vi "Main Tclk.vi"() -> ()   [LabVIEW 2018] (continued)
                        n5203 = local write "Status message"("Scanning FIB vertically to obtain beam profile" ("Status message")) -> ()
                        n5204 = Get Date/Time In Seconds() -> (seconds since 1Jan1904=w4280:timestamp)
                        n5205 = To Double Precision Float(number=w4280) -> (double precision float=w4279:dbl)
                        n5206 = property on="Measurements" class="WFChart (strict)"("History Data"=dbl[][] [], "XScale.Offset"=w4279) -> ()  [unwired: 2 in, 2 out]
                        n5207 = call "Wait to resume.vi"() -> ()  [unwired: 12 in]
                      }
                      frame #3 {
                        n5208 = local read "Logging status before profiling"() -> (w4306:bool)
                        n5209 = local write "FIB Profile"(FALSE ("FIB Profile")) -> ()
                        n5210 = local write "Enable logging"(w4306) -> ()
                      }
                    }
                  }
                }
              }
            }
          }
          event "Milling para": Value Change {
            n5211 = event-data() -> ()  [unwired: 2 out]
            n5212 = local read "Milling para"() -> (w4322:T35)
            n5213 = local read "FIB"() -> (w4328:bool)
            n5214 = case shown="True" w4328 {
              tunnel: [TRUE ("Origin") FALSE ("Origin")] -> w4329
              tunnel: [0.0 ("Y offset pre (um)") w4345] -> w4327
              frame False {
              }
              frame True {
                n5215 = local read "Y offset pre (um)"() -> (w4345:dbl)
              }
            }
            n5216 = Unbundle By Name(w4322) -> ("X size (um)"=w4337:sgl, "Z size (um)"=w4336:sgl, "Z-step (nm)"=w4308:dbl)
            n5217 = local write "SW error warning armed"(FALSE ("SW error warning armed")) -> ()
            n5218 = local write "Cycle time array"(u32[] [] ("Cycle time array")) -> ()
            n5219 = local write "Cycle time est offset array"(i16[] [] ("Cycle time array")) -> ()
            n5220 = expression code="x/1e3"(w4308) -> (w4334:dbl)
            n5221 = control-ref of="FIB Image"() -> (w4330:refnum<vi>)
            n5222 = local read "FIB Scan Parameters"() -> (w4321:T32)
            n5223 = local read "FIB Options"() -> (w4320:T33)
            n5224 = shared-variable ".\\Zeiss Library.lvlib\\Milling Z Voltage RT"() -> (w4319:sgl)  [unwired: 1 in, 1 out]
            n5225 = expression code="log2( x/0.1)"(w4337) -> (w4339:sgl)
            n5226 = Round Toward +Infinity(x=w4339) -> (ceil(x): smallest int >= x=w4341:sgl)
            n5227 = Scale By Power Of 2(n=w4341, x=ext 1.0) -> (x*2^n=w4338:ext)
            n5228 = Divide(x=w4336, y=w4334) -> (x/y=w4342:dbl)
            n5229 = Round To Nearest(number=w4342) -> (nearest integer value=w4331:dbl)
            n5230 = local read "Milling para"() -> (w4333:T35)
            n5231 = Increment(x=w4331) -> (x+1=w4332:dbl)
            n5232 = Multiply(x=w4331, y=w4334) -> (x*y=w4335:dbl)
            n5233 = Bundle By Name(cluster=w4333, "X resolution"=w4338, "Z resolution"=w4332, "Z size (um)"=w4335) -> (w4312:T35)
            n5234 = call "FIB image draw milling.vi"("Milling Z Voltage"=w4319, "Milling para"=w4312, "Z offset pre (um)"=w4327, "FIB Options"=w4320, "FIB Scan Parameters"=w4321, "Origin"=w4329, "Image reference"=w4330) -> ("X size factor"=w4310:dbl, "Trapezoidal"=w4309:cluster{"X":i16, "Y":i16}[])  [unwired: 3 in]
            n5235 = local write "Trapezoidal"(w4309) -> ()
            n5236 = control-ref of="Post Image"() -> (w4326:refnum<vi>)
            n5237 = local read "FIB Zoom Parameters"() -> (w4318:T34)
            n5238 = local write "Milling para"(w4312) -> ()
            n5239 = local read "X offset pre (um)"() -> (w4324:dbl)
            n5240 = local read "Y offset pre (um)"() -> (w4323:dbl)
            n5241 = call "FIB zoom image draw milling.vi"("Milling Z voltage"=w4319, "Milling para"=w4312, "Z offset pre (um)"=w4323, "X offset pre (um)"=w4324, "FIB Zoom Parameters"=w4318, "FIB Options"=w4320, "FIB Scan Parameters"=w4321, "Pre image"=FALSE, "Image reference"=w4326) -> ()  [unwired: 3 in]
            n5242 = Unbundle By Name(w4312) -> ("Line milling time (s)"=w4313:sgl, "Lines auto pause"=w4314:u16)
            n5243 = Compound Arithmetic op=MULTIPLY(w4313, w4314, w4310) -> (w4311:dbl)
            n5244 = local write "Milling time (s)"(w4311) -> ()
          }
          event "Milling para.Z-step (nm)": Value Change {
            n5245 = event-data() -> ()  [unwired: 7 out]
            n5246 = local read "Milling para"() -> (w4350:T35)
            n5247 = local read "FIB"() -> (w4351:bool)
            n5248 = case shown="True" w4351 {
              tunnel: [TRUE ("Origin") FALSE ("Origin")] -> w4352
              tunnel: [0.0 ("Y offset pre (um)") w4372] -> w4349
              frame False {
              }
              frame True {
                n5249 = local read "Y offset pre (um)"() -> (w4372:dbl)
              }
            }
            n5250 = Unbundle By Name(w4350) -> ("X size (um)"=w4363:sgl, "Z size (um)"=w4362:sgl, "Z-step (nm)"=w4347:dbl)
            n5251 = expression code="x/1e3"(w4347) -> (w4360:dbl)
            n5252 = control-ref of="FIB Image"() -> (w4356:refnum<vi>)
            n5253 = local read "FIB Scan Parameters"() -> (w4355:T32)
            n5254 = local read "FIB Options"() -> (w4354:T33)
            n5255 = shared-variable ".\\Zeiss Library.lvlib\\Milling Z Voltage RT"() -> (w4353:sgl)  [unwired: 1 in, 1 out]
            n5256 = expression code="log2( x/0.1)"(w4363) -> (w4365:sgl)
            n5257 = Round Toward +Infinity(x=w4365) -> (ceil(x): smallest int >= x=w4367:sgl)
            n5258 = call "FIB image draw milling.vi"("Milling Z Voltage"=w4353, "Milling para"=w4350, "Z offset pre (um)"=w4349, "FIB Options"=w4354, "FIB Scan Parameters"=w4355, "Origin"=w4352, "Image reference"=w4356) -> ()  [unwired: 3 in, 2 out]
            n5259 = Scale By Power Of 2(n=w4367, x=ext 1.0) -> (x*2^n=w4364:ext)
            n5260 = Divide(x=w4362, y=w4360) -> (x/y=w4368:dbl)
            n5261 = Round To Nearest(number=w4368) -> (nearest integer value=w4357:dbl)
            n5262 = local read "Milling para"() -> (w4359:T35)
            n5263 = Increment(x=w4357) -> (x+1=w4358:dbl)
            n5264 = Multiply(x=w4357, y=w4360) -> (x*y=w4361:dbl)
            n5265 = Round To Nearest(number=w4361) -> (nearest integer value=w4348:dbl)
            n5266 = Bundle By Name(cluster=w4359, "X resolution"=w4364, "Z resolution"=w4358, "Z size (um)"=w4348) -> (w4369:T35)
            n5267 = local write "Milling para"(w4369) -> ()
          }
          event "Milling para.Mill start from Last": Value Change {
            n5268 = event-data() -> ("NewVal"=w4374:bool)  [unwired: 6 out]
            n5269 = case shown="True" w4374 {
              frame False {
              }
              frame True {
                n5270 = stacked-sequence {
                  frame #0 {
                    n5271 = local read "Last milling snapshot"() -> (w4378:path)
                    n5272 = local read "Last FIB recipe"() -> (w4384:path)
                    n5273 = local read "Re-engage Files"() -> (w4390:path)
                    n5274 = File/Directory Info(path=w4384) -> (path out=w4383:path, error out=w4379:errorcluster)  [unwired: 1 in, 5 out]
                    n5275 = Build Path(base path=w4390, name or relative path="pre.png") -> (appended path=w4388:path)
                    n5276 = File/Directory Info(path=w4378) -> (path out=w4377:path, error out=w4375:errorcluster)  [unwired: 1 in, 5 out]
                    n5277 = Unbundle By Name(w4379) -> ("status"=w4380:bool)
                    n5278 = Unbundle By Name(w4375) -> ("status"=w4376:bool)
                    n5279 = File/Directory Info(path=w4388) -> (error out=w4385:errorcluster)  [unwired: 1 in, 6 out]
                    n5280 = case shown="False" w4376 {
                      tunnel: w4377 -> [w4394 _]
                      tunnel: [w4393 w4396] -> w4387
                      tunnel: w4375 -> [_ w4396]
                      frame False {
                        n5281 = call-poly <vilib>:"Read From XML File.vi"("XML File Path"=w4394) -> ("error out"=w4392:errorcluster, "XML Elements"=w4395:string)  [unwired: 8 in, 1 out]
                        n5282 = Unflatten From XML(xml string=w4395, type=T46 {"Timestamp"=timestamp(0 s since 1904-01-01), "Milling Z voltage"=0.0, "FIB slice #"=0, "Pause for reheat"=FALSE, "Last good FI"=0.0, "Focus index"=0.0, "SEM max FOV"=0.0, "Remaining X shift frames"=0, "Remaining Y shift frames"=0} ("output cluster"), error in (no error)=w4392) -> (error out=w4393:errorcluster)  [unwired: 1 out]
                      }
                      frame True {
                      }
                    }
                    n5283 = case shown="False" w4380 {
                      tunnel: [w4398 w4400] -> w4386
                      tunnel: w4383 -> [w4397 _]
                      tunnel: w4379 -> [_ w4400]
                      frame False {
                        n5284 = call "Recipe read write.vi"("Write"=FALSE, "Recipe path"=w4397) -> ("error out"=w4398:errorcluster)  [unwired: 6 in, 3 out]
                      }
                      frame True {
                      }
                    }
                    n5285 = Merge Errors(w4387, w4386, w4385) -> (w4381:errorcluster)
                    n5286 = Unbundle By Name(w4381) -> ("status"=w4382:bool)
                    n5287 = local write "error out"(w4381) -> ()
                    n5288 = case shown="True" w4382 {
                      frame False {
                      }
                      frame True {
                        n5289 = local read "Milling para"() -> (w4403:T35)
                        n5290 = Two Button Dialog(message="Files needed for resume do not exist or are corrupted\nLoad information from the last good data file (*.dat)?") -> (T button?=w4401:bool)  [unwired: 2 in]
                        "dat to csv and xml" <- w4401
                        n5291 = Bundle By Name(cluster=w4403, "Mill start from Last"=w4401) -> (w4402:T35)
                        n5292 = local write "Milling para"(w4402) -> ()
                      }
                    }
                  }
                  frame #1 {
                    n5293 = local read "dat to csv and xml"() -> (w4405:bool)
                    n5294 = case shown="True" w4405 {
                      frame False {
                      }
                      frame True {
                        n5295 = call "File Dialog4"("start path"=path "E:/Images", "prompt"="Select the last good .dat file", "pattern (all files)"="*.dat" ("pattern label"), "pattern label"="Data file") -> ("selected path"=w4408:path, "cancelled"=w4406:bool, "error out"=w4411:errorcluster)  [unwired: 8 in, 1 out]
                        n5296 = local write "Read recipe path"(w4408) -> ()
                        n5297 = local write "error out"(w4411) -> ()
                        n5298 = case shown="True" w4406 {
                          frame False {
                            n5299 = local write "Load recipe"(TRUE ("Load recipe")) -> ()
                          }
                          frame True {
                            n5300 = local read "Milling para"() -> (w4414:T35)
                            n5301 = Bundle By Name(cluster=w4414, "Mill start from Last"=FALSE) -> (w4416:T35)
                            n5302 = local write "Milling para"(w4416) -> ()
                          }
                        }
                      }
                    }
                  }
                  frame #2 {
                    n5303 = local read "Milling para"() -> (w4418:T35)
                    n5304 = Unbundle By Name(w4418) -> ("Mill start from Last"=w4417:bool)
                    n5305 = case shown="True" w4417 {
                      frame False {
                      }
                      frame True {
                        n5306 = One Button Dialog(message="Resume from the last recipe and milling position ") -> ()  [unwired: 1 in, 1 out]
                      }
                    }
                  }
                }
              }
            }
          }
          event "Milling para.FIB PID reset": Value Change {
            n5307 = event-data() -> ("NewVal"=w4420:bool)  [unwired: 2 out]
            n5308 = shared-variable ".\\Zeiss Library.lvlib\\FIB PID reset"(w4420) -> ()  [unwired: 1 in, 1 out]
          }
          event "Milling para.FIB PID target": Value Change {
            w4421 = FALSE ("FIB CL current alarm")
            n5309 = event-data() -> ()  [unwired: 7 out]
            n5310 = local write "Continued fine milling frames"(0 ("Continued fine milling frames")) -> ()
            n5311 = local read "Alert Settings"() -> (w4424:T36)
            n5312 = Bundle By Name(cluster=w4424, "FIB CL current alarm"=w4421, "Milling Z voltage alarm"=w4421) -> (w4423:T36)
            n5313 = local write "Alert Settings"(w4423) -> ()
          }
          event "Pre image": Value Change {
            n5314 = event-data() -> ("NewVal"=w4425:bool)  [unwired: 2 out]
            n5315 = case shown="True" w4425 {
              frame False {
                n5316 = local write "Status message"("standby" ("Status message")) -> ()
                n5317 = shared-variable "My Computer\\Zeiss Library.lvlib\\Realtime Imaging stop"(TRUE ("Unfreeze")) -> ()  [unwired: 1 in, 1 out]
              }
              frame True {
                n5318 = stacked-sequence {
                  frame #0 {
                    n5319 = local read "FIB HW Config"() -> (w4436:T23)
                    n5320 = local read "FIB HW Config"() -> (w4433:T23)
                    n5321 = local write "Status message"("FIB Pre Imaging" ("Status message")) -> ()
                    n5322 = Unbundle By Name(w4436) -> ("Beam blank"=w4435:tag)
                    n5323 = Unbundle By Name(w4433) -> ("FIB Ext Scan"=w4431:tag)
                    n5324 = local read "Api"() -> (w4428:refnum<k7>)
                    n5325 = call "FIB beam blank.vi"("ActiveX Container"=w4428, "Beam blanked"=TRUE, "lines"=w4435) -> ()  [unwired: 2 in, 1 out]
                    n5326 = call "FIB ext scan.vi"("Ext on"=TRUE ("data"), "FIB Ext Scan"=w4431) -> ()  [unwired: 9 in, 1 out]
                    n5327 = local write "Image Tabs"(T37."FIB Milling Offset after Pause" ("Image Tabs")) -> ()
                  }
                  frame #1 {
                    n5328 = local read "Machine Type"() -> (w4437:u8)
                    n5329 = case shown="1" w4437 {
                      frame 0, Default {
                      }
                      frame 1 {
                        w4440 = TRUE ("Close session")
                        n5330 = local read "COM port"() -> (w4442:refnum<visa-resource-name>)
                        n5331 = call "Remcon32 command.vi"("Initialization"=w4440, "SEM command"="edx 1", "COM port in"=w4442) -> ("COM port out"=w4441:refnum<visa-resource-name>)  [unwired: 5 in, 3 out]
                        n5332 = call "FIB mode.vi"("Close session"=w4440, "Iterations"=u32 3, "FIB mode"=T10."FIB", "COM port in"=w4441) -> ()  [unwired: 6 in, 2 out]
                      }
                    }
                  }
                  frame #2 {
                    n5333 = shared-variable ".\\Zeiss Library.lvlib\\Milling Z Voltage RT"() -> (w4445:sgl)  [unwired: 1 in, 1 out]
                    n5334 = local read "FIB Options"() -> (w4448:T33)
                    n5335 = local read "FIB Scan Parameters"() -> (w4452:T32)
                    n5336 = property on="Pre Image" class="IntGraph (strict)"() -> ("Width"=w4461:u32, "Height"=w4460:u32)  [unwired: 2 in, 2 out]
                    n5337 = local read "FIB Options"() -> (w4468:T33)
                    n5338 = local read "Milling para"() -> (w4451:T35)
                    n5339 = local read "FIB Scan Parameters"() -> (w4474:T32)
                    n5340 = expression code="x/1000"("FIB Y zoom pixel (nm)") -> (w4462:dbl)
                    n5341 = Decrement(x=w4460) -> (x-1=w4459:u32)
                    n5342 = Unbundle By Name(w4448) -> ("Flip z"=w4447:bool)
                    n5343 = Unbundle By Name(w4468) -> ("Flip x"=w4464:bool)
                    n5344 = Unbundle By Name(w4451) -> ("X offset (um)"=w4480:sgl, "X center (um)"=w4479:sgl, "FIB FOV (um)"=w4450:sgl)
                    n5345 = Multiply(x=w4462, y=w4459) -> (x*y=w4458:dbl)
                    "FIB Y zoom size (um)" <- w4458
                    n5346 = Unbundle By Name(w4452) -> ("Z size (V)"=w4453:dbl)
                    n5347 = Unbundle By Name(w4474) -> ("X size (V)"=w4469:dbl)
                    n5348 = Negate(x=w4445) -> (-x=w4446:sgl)
                    n5349 = Add(x=w4480, y=w4479) -> (x+y=w4481:sgl)
                    n5350 = Select(t=w4446, s=w4447, f=w4445) -> (s? t:f=w4444:sgl)
                    n5351 = Divide(x=w4444, y=w4453) -> (x/y=w4454:dbl)
                    n5352 = Multiply(x=w4454, y=w4450) -> (x*y=w4455:dbl)
                    n5353 = shared-variable ".\\Zeiss Library.lvlib\\Milling Z Voltage RT"() -> (w4477:sgl)  [unwired: 1 in, 1 out]
                    n5354 = call "Milling parameter to trapezoidal shape.vi"("Y location (um)"=w4455, "Milling para"=w4451) -> ("X size (um) @ Y"=w4449:dbl)  [unwired: 5 in, 4 out]
                    n5355 = expression code="x*1.2"(w4449) -> (w4456:dbl)
                    "FIB X zoom size (um)" <- w4456
                    n5356 = Divide(x=w4481, y=w4450) -> (x/y=w4470:sgl)
                    n5357 = Divide(x=w4456, y=w4450) -> (x/y=w4473:dbl)
                    n5358 = Multiply(x=w4470, y=w4469) -> (x*y=w4466:dbl)
                    n5359 = Multiply(x=w4473, y=w4469) -> (x*y=w4457:dbl)
                    n5360 = Multiply(x=w4469, y=w4458) -> (x*y=w4472:dbl)
                    n5361 = Negate(x=w4466) -> (-x=w4467:dbl)
                    n5362 = Divide(x=w4472, y=w4450) -> (x/y=w4471:dbl)
                    n5363 = Select(t=w4467, s=w4464, f=w4466) -> (s? t:f=w4465:dbl)
                    n5364 = local read "FIB Zoom Parameters"() -> (w4483:T34)
                    n5365 = Bundle By Name(cluster=w4483, "X resolution"=w4461, "Y resolution"=w4459, "X center"=w4465, "X size (V)"=w4457, "Y center"=w4477, "Y size (V)"=w4471, "Frame line rampdown ratio"=-0.1, "Scan rate (Hz)"=u32 200000, "Oversampling"=u16 20) -> (w4482:T34)
                    n5366 = local write "FIB Zoom Parameters"(w4482) -> ()
                  }
                  frame #3 {
                    n5367 = Wait (ms)(milliseconds to wait=u32 200) -> ()  [unwired: 1 out]
                  }
                  frame #4 {
                    w4487 = TRUE ("As subVi")
                    n5368 = local read "FIB HW Config"() -> (w4488:T23)
                    n5369 = local read "FIB Options"() -> (w4489:T33)
                    n5370 = local read "Api"() -> (w4485:refnum<k7>)
                    n5371 = call "FIB realtime imaging PXIe-6124.vi"("HW Config"=w4488, "Options"=w4489, "Single scan"=w4487, "Scan Para"="FIB Zoom Parameters", "As subVi"=w4487, "ActiveX Container"=w4485) -> ()  [unwired: 3 in, 2 out]
                  }
                  frame #5 {
                    n5372 = Wait (ms)(milliseconds to wait=u32 100) -> ()  [unwired: 1 out]
                    n5373 = local read "Milling para"() -> (w4495:T35)
                    n5374 = local read "FIB Zoom Parameters"() -> (w4490:T34)
                    n5375 = control-ref of="Pre Image"() -> (w4498:refnum<vi>)
                    n5376 = local read "FIB Scan Parameters"() -> (w4493:T32)
                    n5377 = local read "FIB Options"() -> (w4492:T33)
                    n5378 = shared-variable ".\\Zeiss Library.lvlib\\Milling Z Voltage RT"() -> (w4491:sgl)  [unwired: 1 in, 1 out]
                    n5379 = call "FIB zoom image draw milling.vi"("Milling Z voltage"=w4491, "Milling para"=w4495, "FIB Zoom Parameters"=w4490, "FIB Options"=w4492, "FIB Scan Parameters"=w4493, "Pre image"=TRUE, "Image reference"=w4498) -> ()  [unwired: 5 in]
                    n5380 = Unbundle By Name(w4495) -> ("X offset (um)"=→"X offset pre (um)":sgl, "Z offset (um)"=→"Y offset pre (um)":sgl)
                  }
                  frame #6 {
                    n5381 = local read "Pre Image"() -> (w4500:i16[][])
                    n5382 = Array Size(array=w4500) -> (size(s)=w4501:i32[])
                    n5383 = local write "Pre image"(FALSE ("Pre image")) -> ()
                    n5384 = local write "Status message"("standby" ("Status message")) -> ()
                    n5385 = Add Array Elements(numeric array=w4501) -> (sum=w4502:i32)
                    n5386 = Not Equal To 0?(x=w4502) -> (x != 0?=w4503:bool)
                    n5387 = case shown="True" w4503 {
                      tunnel: w4500 -> [_ w4508]
                      frame False {
                      }
                      frame True {
                        n5388 = local read "Last FIB zoom pre image"() -> (w4510:path)
                        n5389 = call "16bit Image Normalization.vi"("Transpose"=FALSE, "Input image"=w4508) -> ("Normalized image"=w4507:u8[][])  [unwired: 5 in, 4 out]
                        n5390 = call <vilib>:"Flatten Pixmap.vi"("colors"=u32[] [16777222, 65793, 131586, 197379, 263172, 328965, 394758, 460551, 526344, 592137, 657930, 723723, 789516, 855309, 921102, 986895, 1052688, 1118481, 1184274, 1250067, 1315860, 1381653, 1447446, 1513239, 1579032, 1644825, 1710618, 1776411, 1842204, 1907997, 1973790, 2039583, 2105376, 2171169, 2236962, 2302755, 2368548, 2434341, 2500134, 2565927, 2631720, 2697513, 2763306, 2829099, 2894892, 2960685, 3026478, 3092271, 3158064, 3223857, 3289650, 3355443, 3421236, 3487029, 3552822, 3618615, 3684408, 3750201, 3815994, 3881787, 3947580, 4013373, 4079166, 4144959, 4210752, 4276545, 4342338, 4408131, 4473924, 4539717, 4605510, 4671303, 4737096, 4802889, 4868682, 4934475, 5000268, 5066061, 5131854, 5197647, 5263440, 5329233, 5395026, 5460819, 5526612, 5592405, 5658198, 5723991, 5789784, 5855577, 5921370, 5987163, 6052956, 6118749, 6184542, 6250335, 6316128, 6381921, 6447714, 6513507, 6579300, 6645093, 6710886, 6776679, 6842472, 6908265, 6974058, 7039851, 7105644, 7171437, 7237230, 7303023, 7368816, 7434609, 7500402, 7566195, 7631988, 7697781, 7763574, 7829367, 7895160, 7960953, 8026746, 8092539, 8158332, 8224125, 8289918, 8355711, 8421504, 8487297, 8553090, 8618883, 8684676, 8750469, 8816262, 8882055, 8947848, 9013641, 9079434, 9145227, 9211020, 9276813, 9342606, 9408399, 9474192, 9539985, 9605778, 9671571, 9737364, 9803157, 9868950, 9934743, 10000536, 10066329, 10132122, 10197915, 10263708, 10329501, 10395294, 10461087, 10526880, 10592673, 10658466, 10724259, 10790052, 10855845, 10921638, 10987431, 11053224, 11119017, 11184810, 11250603, 11316396, 11382189, 11447982, 11513775, 11579568, 11645361, 11711154, 11776947, 11842740, 11908533, 11974326, 12040119, 12105912, 12171705, 12237498, 12303291, 12369084, 12434877, 12500670, 12566463, 12632256, 12698049, 12763842, 12829635, 12895428, 12961221, 13027014, 13092807, 13158600, 13224393, 13290186, 13355979, 13421772, 13487565, 13553358, 13619151, 13684944, 13750737, 13816530, 13882323, 13948116, 14013909, 14079702, 14145495, 14211288, 14277081, 14342874, 14408667, 14474460, 14540253, 14606046, 14671839, 14737632, 14803425, 14869218, 14935011, 15000804, 15066597, 15132390, 15198183, 15263976, 15329769, 15395562, 15461355, 15527148, 15592941, 15658734, 15724527, 15790320, 15856113, 15921906, 15987699, 16053492, 16119285, 16185078, 16250871, 16316664, 16382457, 16448250, 16514043, 16579836, 16645629, 16711422, 16448250] ("256 gray scale"), "8-bit pixmap"=w4507) -> ("image data"=w4509:T52)  [unwired: 4 in, 5 out]
                        n5391 = call <vilib>:"Write PNG File.vi"("image data"=w4509, "path to PNG file"=w4510) -> ()  [unwired: 1 in, 9 out]
                      }
                    }
                  }
                }
              }
            }
          }
          event "Post image": Value Change {
            n5392 = event-data() -> ("NewVal"=w4512:bool)  [unwired: 2 out]
            n5393 = case shown="True" w4512 {
              frame False {
                n5394 = local write "Status message"("standby" ("Status message")) -> ()
                n5395 = shared-variable "My Computer\\Zeiss Library.lvlib\\Realtime Imaging stop"(TRUE ("Unfreeze")) -> ()  [unwired: 1 in, 1 out]
              }
              frame True {
                n5396 = stacked-sequence {
                  frame #0 {
                    n5397 = local read "FIB HW Config"() -> (w4523:T23)
                    n5398 = local read "FIB HW Config"() -> (w4520:T23)
                    n5399 = local write "Status message"("FIB Post Imaging" ("Status message")) -> ()
                    n5400 = Unbundle By Name(w4523) -> ("Beam blank"=w4522:tag)
                    n5401 = Unbundle By Name(w4520) -> ("FIB Ext Scan"=w4518:tag)
                    n5402 = local read "Api"() -> (w4515:refnum<k7>)
                    n5403 = call "FIB beam blank.vi"("ActiveX Container"=w4515, "Beam blanked"=TRUE, "lines"=w4522) -> ()  [unwired: 2 in, 1 out]
                    n5404 = call "FIB ext scan.vi"("Ext on"=TRUE ("data"), "FIB Ext Scan"=w4518) -> ()  [unwired: 9 in, 1 out]
                    n5405 = local write "Image Tabs"(T37."FIB Milling Offset after Pause" ("Image Tabs")) -> ()
                  }
                  frame #1 {
                    n5406 = local read "Machine Type"() -> (w4524:u8)
                    n5407 = case shown="1" w4524 {
                      frame 0, Default {
                      }
                      frame 1 {
                        w4527 = TRUE ("Close session")
                        n5408 = local read "COM port"() -> (w4529:refnum<visa-resource-name>)
                        n5409 = call "Remcon32 command.vi"("Initialization"=w4527, "SEM command"="edx 1", "COM port in"=w4529) -> ("COM port out"=w4528:refnum<visa-resource-name>)  [unwired: 5 in, 3 out]
                        n5410 = call "FIB mode.vi"("Close session"=w4527, "Iterations"=u32 3, "FIB mode"=T10."FIB", "COM port in"=w4528) -> ()  [unwired: 6 in, 2 out]
                      }
                    }
                  }
                  frame #2 {
                    n5411 = local read "FIB Y zoom pixel (nm)"() -> (w4551:dbl)
                    n5412 = property on="Pre Image" class="IntGraph (strict)"() -> ("Height"=w4550:u32)  [unwired: 2 in, 2 out]
                    n5413 = local read "FIB Scan Parameters"() -> (w4547:T32)
                    n5414 = local read "Milling para"() -> (w4548:T35)
                    n5415 = local read "FIB Zoom Parameters"() -> (w4533:T34)
                    n5416 = shared-variable ".\\Zeiss Library.lvlib\\Milling Z Voltage RT"() -> (w4532:sgl)  [unwired: 1 in, 1 out]
                    n5417 = Decrement(x=w4550) -> (x-1=w4541:u32)
                    n5418 = Unbundle By Name(w4548) -> ("FIB FOV (um)"=w4549:sgl)
                    n5419 = Unbundle By Name(w4547) -> ("X size (V)"=w4546:dbl)
                    n5420 = expression code="x/1000"(w4551) -> (w4542:dbl)
                    n5421 = Unbundle By Name(w4533) -> ("Y size (V)"=w4538:dbl)
                    n5422 = Bundle By Name(cluster=w4533, "Y center"=w4532) -> (w4531:T34)
                    n5423 = Multiply(x=w4541, y=w4546) -> (x*y=w4545:dbl)
                    n5424 = Divide(x=w4545, y=w4549) -> (x/y=w4544:dbl)
                    n5425 = local write "FIB Zoom Parameters"(w4531) -> ()
                    n5426 = Divide(x=w4538, y=w4544) -> (x/y=w4543:dbl)
                    n5427 = Multiply(x=w4542, y=w4544) -> (x*y=w4539:dbl)
                    n5428 = Subtract(x=w4539, y=w4538) -> (x-y=w4535:dbl)
                    n5429 = Multiply(x=w4542, y=w4541) -> (x*y=w4540:dbl)
                    n5430 = Absolute Value(x=w4535) -> (abs(x)=w4534:dbl)
                    n5431 = Greater?(x=w4534, y=0.0001) -> (0:w4537:bool)
                    n5432 = case shown="True" w4537 {
                      tunnel: w4539 -> [_ w4557]
                      tunnel: w4543 -> [_ w4554]
                      tunnel: w4540 -> [_ w4552]
                      frame False {
                      }
                      frame True {
                        n5433 = expression code="x*1000"(w4554) -> (w4553:dbl)
                        n5434 = Two Button Dialog(message="Y pixel was modified since the last pre image was taken", 1:"Continue with new value" ("T button name (\"OK\")"), 2:"Use old value" ("T button name (\"OK\")")) -> (T button?=w4558:bool)
                        n5435 = case shown="True" w4558 {
                          tunnel: w4557 -> [w4561 _]
                          tunnel: w4553 -> [_ w4564]
                          tunnel: w4552 -> [w4560 _]
                          frame False {
                            n5436 = local read "FIB Zoom Parameters"() -> (w4563:T34)
                            n5437 = Bundle By Name(cluster=w4563, "Y size (V)"=w4561) -> (w4562:T34)
                            n5438 = local write "FIB Zoom Parameters"(w4562) -> ()
                            n5439 = local write "FIB Y zoom size (um)"(w4560) -> ()
                          }
                          frame True {
                            n5440 = local write "FIB Y zoom pixel (nm)"(w4564) -> ()
                          }
                        }
                      }
                    }
                  }
                  frame #3 {
                    w4567 = TRUE ("As subVi")
                    n5441 = local read "FIB HW Config"() -> (w4568:T23)
                    n5442 = local read "FIB Options"() -> (w4569:T33)
                    n5443 = local read "FIB Zoom Parameters"() -> (w4566:T34)
                    n5444 = local read "Api"() -> (w4565:refnum<k7>)
                    n5445 = call "FIB realtime imaging PXIe-6124.vi"("HW Config"=w4568, "Options"=w4569, "Single scan"=w4567, "Scan Para"=w4566, "As subVi"=w4567, "ActiveX Container"=w4565) -> ()  [unwired: 3 in, 2 out]
                  }
                  frame #4 {
                    n5446 = Wait (ms)(milliseconds to wait=u32 100) -> ()  [unwired: 1 out]
                  }
                  frame #5 {
                    n5447 = local read "FIB Zoom Parameters"() -> (w4596:T34)
                    n5448 = local read "X offset pre (um)"() -> (w4572:dbl)
                    n5449 = local read "Y offset pre (um)"() -> (w4571:dbl)
                    n5450 = local read "Post Image"() -> (w4585:i16[][])
                    n5451 = local read "Pre Image"() -> (w4584:i16[][])
                    n5452 = call "Image Alignment.vi"("Image 2"=w4584, "Image 1"=w4585) -> ("Y shift"=w4588:i32, "X shift"=w4593:i32)  [unwired: 7 in, 1 out]
                    n5453 = Unbundle By Name(w4596) -> ("X resolution"=w4592:u32, "Y resolution"=w4587:u32, "X size (V)"=w4591:dbl, "Y size (V)"=w4586:dbl)
                    n5454 = Divide(x=w4593, y=w4592) -> (x/y=w4589:dbl)
                    n5455 = Divide(x=w4588, y=w4587) -> (x/y=w4590:dbl)
                    n5456 = local read "Milling para"() -> (w4595:T35)
                    n5457 = local read "FIB Scan Parameters"() -> (w4594:T32)
                    n5458 = Multiply(x=w4589, y=w4591) -> (x*y=w4580:dbl)
                    n5459 = Multiply(x=w4590, y=w4586) -> (x*y=w4581:dbl)
                    n5460 = Unbundle By Name(w4595) -> ("FIB FOV (um)"=w4583:sgl)
                    n5461 = Unbundle By Name(w4594) -> ("X size (V)"=w4582:dbl)
                    n5462 = Divide(x=w4583, y=w4582) -> (x/y=w4579:dbl)
                    n5463 = Multiply(x=w4580, y=w4579) -> (x*y=w4576:dbl)
                    n5464 = Multiply(x=w4581, y=w4579) -> (x*y=w4574:dbl)
                    n5465 = Add(x=w4576, y=w4572) -> (x+y=w4575:dbl)
                    n5466 = Add(x=w4574, y=w4571) -> (x+y=w4573:dbl)
                    n5467 = local read "Milling para"() -> (w4578:T35)
                    n5468 = Bundle By Name(cluster=w4578, "X offset (um)"=w4575, "Z offset (um)"=w4573) -> (w4577:T35)
                    n5469 = local write "Milling para"(w4577) -> ()
                  }
                  frame #6 {
                    n5470 = local read "X offset pre (um)"() -> (w4599:dbl)
                    n5471 = local read "Y offset pre (um)"() -> (w4598:dbl)
                    n5472 = local read "Milling para"() -> (w4604:T35)
                    n5473 = local read "FIB Zoom Parameters"() -> (w4597:T34)
                    n5474 = control-ref of="Post Image"() -> (w4605:refnum<vi>)
                    n5475 = local read "FIB Scan Parameters"() -> (w4602:T32)
                    n5476 = local read "FIB Options"() -> (w4601:T33)
                    n5477 = shared-variable ".\\Zeiss Library.lvlib\\Milling Z Voltage RT"() -> (w4600:sgl)  [unwired: 1 in, 1 out]
                    n5478 = call "FIB zoom image draw milling.vi"("Milling Z voltage"=w4600, "Milling para"=w4604, "Z offset pre (um)"=w4598, "X offset pre (um)"=w4599, "FIB Zoom Parameters"=w4597, "FIB Options"=w4601, "FIB Scan Parameters"=w4602, "Pre image"=FALSE, "Image reference"=w4605) -> ()  [unwired: 3 in]
                  }
                  frame #7 {
                    n5479 = local write "Post image"(FALSE ("Pre image")) -> ()
                    n5480 = local write "Status message"("standby" ("Status message")) -> ()
                  }
                }
              }
            }
          }
          event "Hardware Configuration.Save config file": Value Change {
            # "THIS VI WRITES ALL THE HARDWARE CONFIG TAB CONTROLS TO THE .INI FILE."
            n5481 = event-data() -> ()  [unwired: 2 out]
            n5482 = disable-structure shown="Disabled" {
              frame Disabled {
                n5483 = stacked-sequence {
                  frame #0 {
                    n5484 = local read "HW config items"() -> (w4611:string[])
                    n5485 = local read "Hardware Configuration"() -> (w4615:T25)
                    n5486 = local read "Detector Information"() -> (w4616:T8)
                    n5487 = local read "Hardware Configuration"() -> (w4613:T25)
                    n5488 = Unbundle By Name(w4615) -> ("Machine ID"=w4624:string, "Machine Type"=w4630:u8, "SEM Max FOV (um)"=w4617:sgl, "Det min (V)"=w4618:dbl, "Det max (V)"=w4619:dbl)
                    n5489 = Unbundle By Name(w4616) -> ("Brightness A"=w4621:dbl, "Contrast A"=w4620:dbl, "Detector B name"=w4625:string, "Brightness B"=w4622:dbl, "Contrast B"=w4623:dbl)
                    n5490 = Unbundle By Name(w4613) -> ("Configuration file"=w4612:path)
                    n5491 = Build Array(w4617, w4618, w4619, w4621, w4620) -> (w4626:dbl[])
                    n5492 = Build Array(w4622, w4623) -> (w4628:dbl[])
                    n5493 = case shown="2" w4630 {
                      tunnel: ["Feiss" ("Machine ID") "NVision" ("Machine ID") "Jeiss" ("Machine ID")] -> w4631
                      frame 0, Default {
                      }
                      frame 1 {
                      }
                      frame 2 {
                      }
                    }
                    n5494 = for {
                      tunnel: w4626 -> [w4652] mode=indexing
                      tunnel: [w4651] -> w4627 mode=indexing
                      n5495 = Format Into String(w4652) -> (resulting string=w4651:string)  [unwired: 3 in, 1 out]
                    }
                    n5496 = for {
                      tunnel: w4628 -> [w4650] mode=indexing
                      tunnel: [w4649] -> w4629 mode=indexing
                      n5497 = Format Into String(w4650) -> (resulting string=w4649:string)  [unwired: 3 in, 1 out]
                    }
                    n5498 = Build Array (concatenate)(w4624, w4631, w4627, w4625, w4629) -> (w4632:string[])
                    n5499 = for {
                      tunnel: w4611 -> [w4645] mode=indexing
                      tunnel: w4632 -> [w4643] mode=indexing
                      tunnel: [w4642] -> w4614 mode=indexing
                      n5500 = Concatenate Strings(w4645, "," ("string"), w4643) -> (w4642:string)
                    }
                    n5501 = Build Path(name or relative path=w4612) -> (appended path=w4635:path)  [unwired: 1 in]
                    n5502 = Open/Create/Replace File(file path (use dialog)=w4635, operation (0:open)=T49."replace or create with confirmation") -> (refnum out=w4637:refnum<file>, error out=w4638:errorcluster)  [unwired: 1 in, 4 out]
                    n5503 = Set File Position(refnum=w4637, from (0:start)=enum16{"start", "end", "current"}."end", error in=w4638) -> (refnum out=w4639:refnum<file>, error out=w4636:errorcluster)  [unwired: 1 out]
                    n5504 = Write to Text File(file (use dialog)=w4639, text=w4614, error in=w4636) -> (refnum out=w4640:refnum<file>, error out=w4641:errorcluster)  [unwired: 2 out]
                    n5505 = Close File(refnum=w4640, error in=w4641) -> ()  [unwired: 2 out]
                  }
                  frame #1 {
                    n5506 = local read "Hardware Configuration"() -> (w4655:T25)
                    n5507 = Bundle By Name(cluster=w4655, "Save config file"=FALSE) -> (w4654:T25)
                    n5508 = local write "Hardware Configuration"(w4654) -> ()
                  }
                }
              }
              frame Enabled {
              }
            }
            n5509 = local read "Hardware Configuration"() -> (w4610:T25)
            n5510 = Bundle By Name(cluster=w4610, "Save config file"=FALSE) -> (w4609:T25)
            n5511 = local write "Hardware Configuration"(w4609) -> ()
            n5512 = call "Write Config Settings to INI file.vi"("Hardware Configuration"=w4609) -> ()  [unwired: 11 in]
          }
          event "File Information.Save recipe": Value Change {
            n5513 = event-data() -> ()  [unwired: 2 out]
            n5514 = stacked-sequence {
              frame #0 {
              }
              frame #1 {
                n5515 = call "File Dialog"("start path"=path "E:/Recipes", "prompt"="Select an existing recipe to \noverwrite or a directory for \nthe new recipe") -> ("selected path"=w4658:path, "cancelled"=w4660:bool, "error out"=→"error out":errorcluster)  [unwired: 10 in, 1 out]
                n5516 = case shown="False" w4660 {
                  tunnel: w4658 -> [w4667 _]
                  frame False {
                    n5517 = Strip Path(path=w4667) -> (name=w4663:string)  [unwired: 1 out]
                    n5518 = xnode "Match Regular Expression"("input string"=w4663, "regular expression"=".csv") -> ("offset past match"=w4665:i32)  [unwired: 4 in, 4 out]
                    n5519 = Equal?(x=w4665, y=-1) -> (x = y?=w4664:bool)
                    n5520 = case shown="True" w4664 {
                      tunnel: [w4670 w4671] -> w4669
                      tunnel: w4663 -> [w4670 _]
                      frame False {
                      }
                      frame True {
                        n5521 = call "Recipe File Name"() -> ("FIB-SEM recipe YY-MM-DD <user input>.csv"=w4671:string)  [unwired: 17 in, 2 out]
                      }
                    }
                    n5522 = local read "Recipe input"() -> (w4661:T7)
                    n5523 = call "Recipe read write.vi"("Write"=TRUE, "Info"=w4669, "Recipe path"=w4667, "Write input"=w4661) -> ()  [unwired: 4 in, 4 out]
                  }
                  frame True {
                  }
                }
              }
              frame #2 {
                n5524 = Wait (ms)(milliseconds to wait=u32 200) -> ()  [unwired: 1 out]
              }
              frame #3 {
                n5525 = local read "File Information"() -> (w4786:T31)
                n5526 = Bundle By Name(cluster=w4786, "Save recipe"=FALSE ("Save config file")) -> (w4785:T31)
                n5527 = local write "File Information"(w4785) -> ()
              }
            }
          }
          event "File Information.Load recipe": Value Change {
            n5528 = event-data() -> ()  [unwired: 2 out]
            n5529 = stacked-sequence {
              tunnel: [w4790 _ _] -> w4788
              tunnel: w4787 -> [w4789 _ _]
              frame #0 {
                n5530 = call "File Dialog2"("start path"=path "E:/images", "prompt"="Select the recipe", "pattern (all files)"="*.csv;*.dat" ("pattern label"), "pattern label"="Recipe or Data file") -> ("selected path"=w4794:path, "cancelled"=w4795:bool, "error out"=w4796:errorcluster)  [unwired: 8 in, 1 out]
                n5531 = local write "error out"(w4796) -> ()
                n5532 = case shown="False" w4795 {
                  tunnel: w4794 -> [w4799 _]
                  tunnel: [w4798 w4827] -> w4790
                  tunnel: w4789 -> [_ w4827]
                  frame False {
                    n5533 = stacked-sequence {
                      tunnel: w4799 -> [w4801 _ _]
                      tunnel: [_ _ w4826] -> w4798
                      frame #0 {
                        n5534 = local write "Read recipe path"(w4801) -> ()
                        n5535 = Strip Path(path=w4801) -> (name=w4804:string)  [unwired: 1 out]
                        n5536 = Match Pattern(string=w4804, regular expression=".dat") -> (offset past match=w4803:i32)  [unwired: 1 in, 3 out]
                        n5537 = Not Equal?(x=w4803, y=-1) -> (x != y?=w4800:bool)
                        n5538 = case shown="True" w4800 {
                          tunnel: w4801 -> [_ w4823]
                          frame False {
                          }
                          frame True {
                            n5539 = call "Zeiss File Header Tclk.vi"("Write"=FALSE, "Input file path"=w4823) -> ("Ouputs"=w4822:T79)  [unwired: 7 in, 2 out]
                            n5540 = Unbundle By Name(w4822) -> ("SEM parameters"=w4821:T13, "FIB parameters"=w4820:T80, "Data Logging"=w4818:T81)
                            n5541 = Unbundle By Name(w4818) -> ("Temp (F)"=w4817:sgl, "FIB Faraday Cup (nA)"=w4816:sgl, "FIB Specimen I (nA)"=w4815:sgl, "Beam Dump 1 (nA)"=w4814:sgl, "Beam Dump 2 (nA)"=w4807:sgl, "Milling I (nA)"=w4806:sgl, "SEM Specimen I (nA)"=w4809:sgl, "Milling Z voltage (V)"=w4813:sgl, "Focus Index"=w4812:sgl, "FIB slice #"=w4811:u32)
                            n5542 = local write "SEM Parameters"(w4821) -> ()
                            n5543 = local write "FIB Parameters"(w4820) -> ()
                            n5544 = local write "Temp (F)"(w4817) -> ()
                            n5545 = local write "Faraday Cup (nA)"(w4816) -> ()
                            n5546 = local write "Specimen I (nA)"(w4815) -> ()
                            n5547 = local write "Beam Dump 1 (nA)"(w4814) -> ()
                            n5548 = local write "Beam Dump 2 (nA)"(w4807) -> ()
                            n5549 = local write "Milling I (nA)"(w4806) -> ()
                            n5550 = local write "Milling Z voltage (V)"(w4813) -> ()
                            n5551 = local write "Focus Index"(w4812) -> ()
                            n5552 = local write "FIB slice #"(w4811) -> ()
                            n5553 = local read "SEM Status"() -> (w4810:T12)
                            n5554 = Bundle By Name(cluster=w4810, "SEM Spec. I (nA)"=w4809) -> (w4808:T12)
                            n5555 = local write "SEM Status"(w4808) -> ()
                          }
                        }
                      }
                      frame #1 {
                        n5556 = local write "Load recipe"(TRUE ("Load recipe")) -> ()
                        n5557 = Wait (ms)(milliseconds to wait=u32 500) -> ()  [unwired: 1 out]
                      }
                      frame #2 {
                        n5558 = local read "Trapezoidal"() -> (w4826:cluster{"X":i16, "Y":i16}[])
                      }
                    }
                  }
                  frame True {
                  }
                }
              }
              frame #1 {
                n5559 = Wait (ms)(milliseconds to wait=u32 200) -> ()  [unwired: 1 out]
              }
              frame #2 {
                n5560 = local read "File Information"() -> (w4831:T31)
                n5561 = Bundle By Name(cluster=w4831, "Load recipe"=FALSE ("Save config file")) -> (w4830:T31)
                n5562 = local write "File Information"(w4830) -> ()
              }
            }
          }
          event "Clear": Value Change {
            n5563 = event-data() -> ()  [unwired: 7 out]
            n5564 = local read "Sample rate (Hz)"() -> (w4832:dbl)
            n5565 = Get Date/Time In Seconds() -> (seconds since 1Jan1904=w4835:timestamp)
            n5566 = Reciprocal(x=w4832) -> (1/x=w4833:dbl)
            n5567 = To Double Precision Float(number=w4835) -> (double precision float=w4834:dbl)
            n5568 = property on="Measurements" class="WFChart (strict)"("History Data"=dbl[][] [], "XScale.Offset"=w4834, "XScale.Multiplier"=w4833) -> ()  [unwired: 2 in, 2 out]
          }
          event "Alert Settings.Temperature alarm": Value Change {
            n5569 = event-data() -> ("NewVal"=w4837:bool)  [unwired: 6 out]
            n5570 = local write "Temperature warning armed"(w4837) -> ()
          }
          event "Alert Settings.SW error warning": Value Change {
            n5571 = event-data() -> ("NewVal"=w4838:bool)  [unwired: 6 out]
            n5572 = local write "SW error warning armed"(w4838) -> ()
          }
          event "Alert Settings.Focus index warning": Value Change {
            n5573 = event-data() -> ("NewVal"=w4839:bool)  [unwired: 6 out]
            n5574 = local write "Focus index warning armed"(w4839) -> ()
          }
          event "Alert Settings": Value Change {
            n5575 = event-data() -> ()  [unwired: 7 out]
            n5576 = local write "Continued fine milling frames"(-5 ("Continued fine milling frames")) -> ()
          }
          event "Coarse milling": Value Change {
            n5577 = event-data() -> ("NewVal"=w4841:bool)  [unwired: 6 out]
            n5578 = case shown="True" w4841 {
              frame False {
              }
              frame True {
                n5579 = Two Button Dialog(message="Quick settings for coarse milling:\n1. Disable certain alarms\n2. Enable low mag scan for every single high mag\n3. Reset image center and shifts to 0\n4. Reset to single tile\n5. Turn off file upload") -> (T button?=w4842:bool)  [unwired: 2 in]
                n5580 = case shown="True" w4842 {
                  frame False {
                    n5581 = local write "Coarse milling"(FALSE ("Coarse milling")) -> ()
                  }
                  frame True {
                    w4858 = sgl[] [0.0] ("dX (um)")
                    w4859 = u8 1 ("X tiles")
                    w4860 = TRUE ("Low mag scan")
                    w4864 = sgl 0.0 ("X center (um)")
                    w4866 = FALSE ("Upload")
                    n5582 = local read "SEM Scan Parameters"() -> (w4850:T26)
                    n5583 = local read "Low Mag SEM"() -> (w4863:T30)
                    n5584 = Bundle By Name(cluster=w4863, "Low mag scan"=w4860, "Low mag interval"=u32 1, "Show HM box"=w4860) -> (w4862:T30)
                    n5585 = Unbundle By Name(w4850) -> ("X stig"=w4857:sgl[][], "Y stig"=w4856:sgl[][], "X aln"=w4855:sgl[][], "Y aln"=w4854:sgl[][], "WD (mm)"=w4853:sgl[][])
                    n5586 = local write "Low Mag SEM"(w4862) -> ()
                    n5587 = Build Array(w4857, w4856, w4855, w4854, w4853) -> (w4852:sgl[][][])
                    n5588 = for {
                      tunnel: [w4875] -> w4851 mode=indexing
                      workers-P: _ -> [_]
                      tunnel: w4852 -> [w4871] mode=indexing
                      w4874 = 1 ("dimension size")
                      n5589 = Array Size(array=w4871) -> (size(s)=w4873:i32[])
                      n5590 = Multiply Array Elements(1:w4873) -> (0:w4872:i32)
                      n5591 = Reshape Array(w4871, w4872) -> (w4877:sgl[])
                      n5592 = call-poly <vilib>:"Mean.vi"("X"=w4877) -> ("mean"=w4876:dbl)  [unwired: 1 out]
                      n5593 = Initialize Array(w4876, w4874, w4874) -> (w4875:dbl[][])
                    }
                    n5594 = local read "Alert Settings"() -> (w4870:T36)
                    n5595 = Bundle By Name(cluster=w4870, "Specimen @ SEM alarm"=w4866, "FIB CL current alarm"=w4866, "Milling Z voltage alarm"=w4866, "Detector over scale warning"=w4866, "Focus index warning"=w4866) -> (w4869:T36)
                    n5596 = local read "SEM Options"() -> (w4868:T27)
                    n5597 = Bundle By Name(cluster=w4868, "Upload"=w4866) -> (w4867:T27)
                    n5598 = Index Array(array=w4851) -> (element #1=w4849:dbl[][], element #2=w4848:dbl[][], element #3=w4847:dbl[][], element #4=w4846:dbl[][], element #5=w4845:dbl[][])  [unwired: 15 in]
                    n5599 = local write "Alert Settings"(w4869) -> ()
                    n5600 = local write "SEM Options"(w4867) -> ()
